vi "Set Sender.vi"(10 "Sender":refnum<class "Sender.lvclass">, 11 "Setup Msg Strategy in":refnum<class "Setup Msg Strategy.lvclass">) -> (3 "Setup Msg Strategy out":refnum<class "Setup Msg Strategy.lvclass">)   [LabVIEW 2021, in "Setup Msg Strategy.lvlib" / "Setup Msg Strategy.lvclass"]
uses:
  Setup Msg Strategy.lvclass
  Setup Msg Strategy.lvclass/Setup Msg Strategy.ctl
  jettl/Sender/Sender/Sender.lvclass
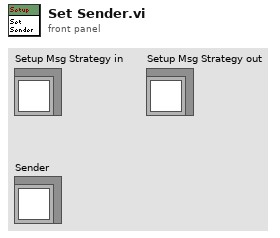
[diagram p1: front panel]
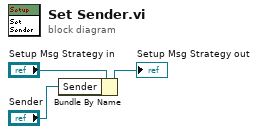
[diagram p0: block diagram]
diagram:
  n1 = Bundle By Name(cluster="Setup Msg Strategy in", "Sender"="Sender") -> (→"Setup Msg Strategy out":refnum<class "Setup Msg Strategy.lvclass">)
